vi "generateTelemetryElevationData.vi"(8 "error in (no error)":errorcluster, 10 "TelemetryElevationData":T1, 11 "UserEvents in":refnum<class "UserEvents.lvclass">) -> (0 "error out":errorcluster, 3 "UserEvents out":refnum<class "UserEvents.lvclass">)   [LabVIEW 2016, in "UserEvents.lvclass"]
uses:
  UserEvents.lvclass
  DataTypes/Topics/TelemetryElevationData.ctl
  DataTypes/Topics/Parts/Timestamp.ctl
  UserEvents.lvclass/UserEvents.ctl
  DataTypes/Topics/M1M3SupportTopics.lvlib
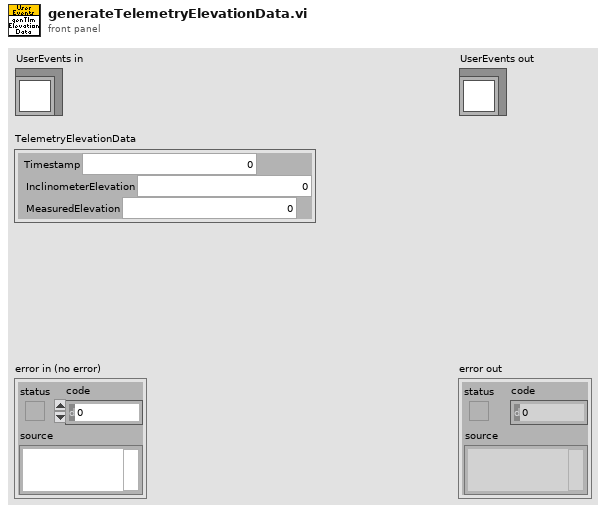
[diagram p1: front panel]
types:
  T1 = typedef "M1M3SupportTopics.lvlib/TelemetryElevationData.ctl" = cluster{"Timestamp":T2, "InclinometerElevation":dbl, "MeasuredElevation":dbl}
  T2 = typedef "M1M3SupportTopics.lvlib/Timestamp.ctl" = dbl
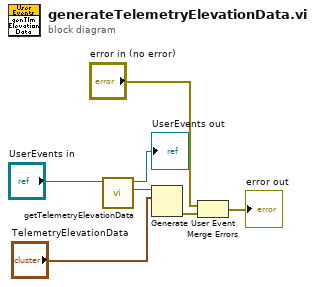
[diagram p0: block diagram]
diagram:
  n1 = call "getTelemetryElevationData.vi"("UserEvents in"="UserEvents in") -> ("TelemetryElevationData"=w7:refnum<user-event>, "UserEvents out"=→"UserEvents out":refnum<class "UserEvents.lvclass">)  [unwired: 9 in]
  n2 = Generate User Event(user event=w7, event data cluster="TelemetryElevationData") -> (error out=w4:errorcluster)  [unwired: 2 in, 1 out]
  n3 = Merge Errors("error in (no error)", w4) -> (→"error out":errorcluster)
